vi "ParseFIFO.vi"(1 "SPC Format":u16(ring)=2 items=["SPC 630 - 32 bit", "SPC 630 - 48 bit", "SPC 830 - 32 bit"], 2 "FIFO rawdata":u16[](array[numeric])) -> (0 "rawdata":T1)   [LabVIEW 2009]
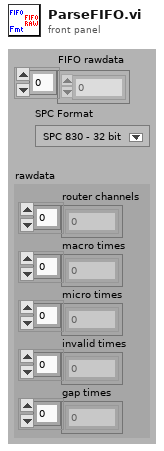
[diagram p1: front panel]
types:
  T1 = cluster{"router channels":u8[], "macro times":u32[], "micro times":u16[], "invalid times":u32[], "gap times":u32[]}
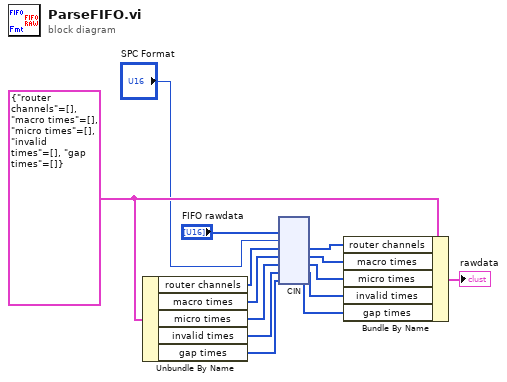
[diagram p0: block diagram]
diagram:
  w8 = T1 {"router channels"=[], "macro times"=[], "micro times"=[], "invalid times"=[], "gap times"=[]}
  n1 = Unbundle By Name(w8) -> ("router channels"=w7:u8[], "macro times"=w6:u32[], "micro times"=w5:u16[], "invalid times"=w4:u32[], "gap times"=w3:u32[])
  n2 = cin("FIFO rawdata", "SPC Format", w7, w6, w5, w4, w3) -> (w13:u8[], w12:u32[], w11:u16[], w10:u32[], w9:u32[])  [unwired: 2 in]
  n3 = Bundle By Name(cluster=w8, "router channels"=w13, "macro times"=w12, "micro times"=w11, "invalid times"=w10, "gap times"=w9) -> (→"rawdata":T1)
